vi "NO_SCAN.vi"(8 "stop":bool, 10 "Address Type":T1=1 items=["Public", "Random"], 11 "COM Bluegiga in":refnum<visa-resource-name>="COM13") -> (0 "Reading":bool, 1 "z":dbl, 3 "Connected":bool)   [LabVIEW 2020]
uses:
  <vilib>/BLE/type_def/connection_status_bundle.ctl
  <vilib>/BLE/type_def/address_type.ctl
panel:
  out "w":dbl
  out "x":dbl
  out "y":dbl
  out "characteristic value":u8[](array[numeric])
  out "MAC Address":string
  in  "Service UUID":string="EF6802009B3549339B1052FFA9740042"
  in  "Characteristic UUID":string="EF6802019B3549339B1052FFA9740042"
  out "Handle table":string[][](array[string])
  out "Connection Status":T2={"MAC Address"="", "cnx handle"=0, "cnx flags"=0, "Address Type"=125, "Connection Interval (ms)"=125, "Timeout(ms)"=125, "Latency"=0, "bonding handle"=0} {"Address Type" items=["Public", "Random"]}
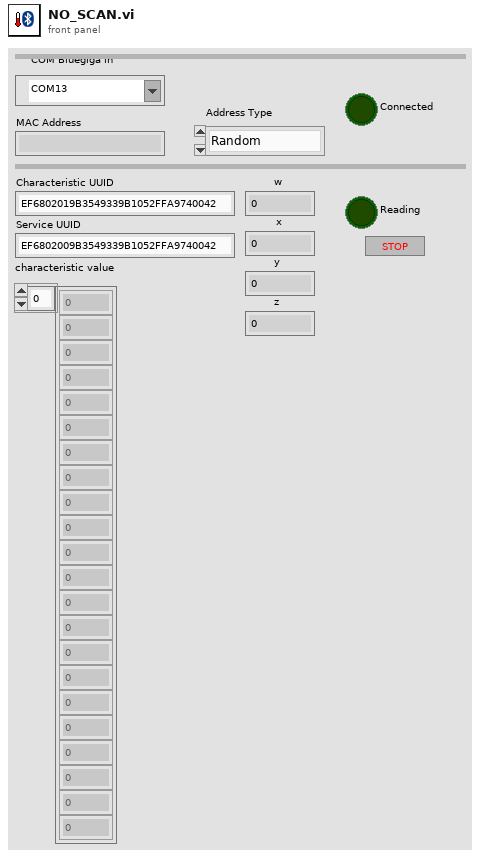
[diagram p1: front panel]
types:
  T1 = typedef "address_type.ctl" = u8
  T2 = typedef "connection_status_bundle.ctl" = cluster{"MAC Address":string, "cnx handle":u8, "cnx flags":u8, "Address Type":T1, "Connection Interval (ms)":u16, "Timeout(ms)":u16, "Latency":u16, "bonding handle":u8}
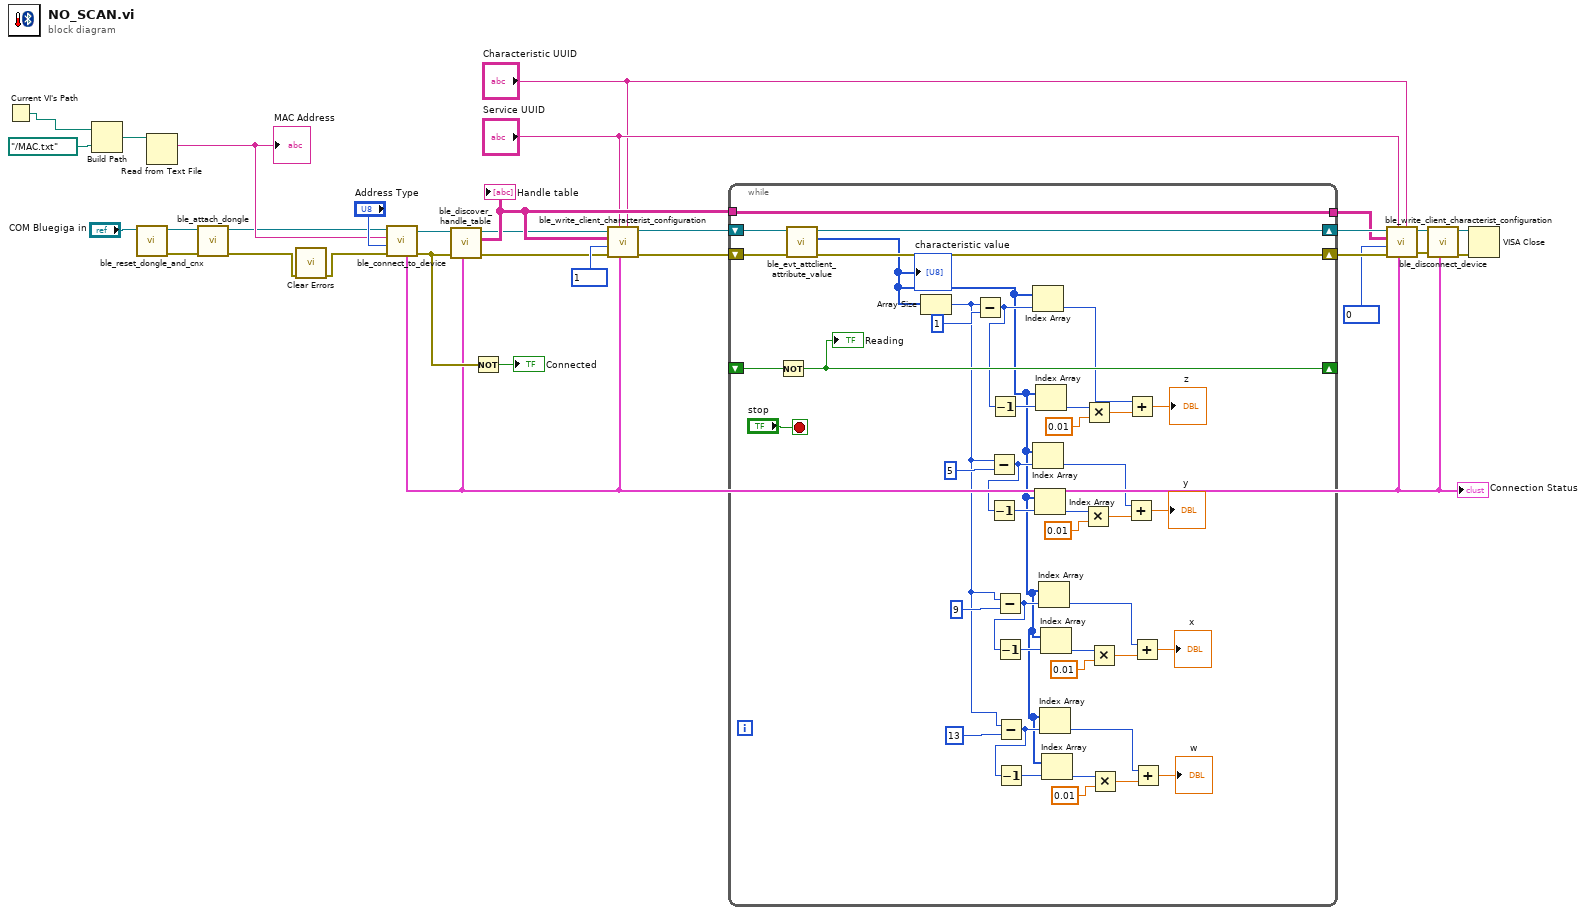
[diagram p0: block diagram]
diagram:
  n1 = Current VI's Path() -> (path=w4:path)
  n2 = Build Path(base path=w4, name or relative path=path "../MAC.txt") -> (appended path=w5:path)
  n3 = call <vilib>:"ble_reset_dongle_and_cnx.vi"("COM Bluegiga in"="COM Bluegiga in") -> ("error out"=w29:errorcluster, "COM Bluegiga out"=w27:refnum<visa-resource-name>)  [unwired: 9 in]
  n4 = Read from Text File(file (use dialog)=w5) -> (text=w7:string)  [unwired: 3 in, 3 out]
  "MAC Address" <- w7
  n5 = call <vilib>:"ble_attach_dongle.vi"("error in (no error)"=w29, "COM Bluegiga in"=w27) -> ("error out"=w2:errorcluster, "COM Bluegiga out"=w3:refnum<visa-resource-name>)  [unwired: 8 in]
  n6 = call <vilib>:"Clear Errors.vi"("error in (no error)"=w2) -> ("error out"=w9:errorcluster)  [unwired: 5 in, 1 out]
  n7 = call <vilib>:"ble_connect_to_device.vi"("Address Type"="Address Type", "error in (no error)"=w9, "MAC Address"=w7, "COM Bluegiga in"=w3) -> ("error out"=w25:errorcluster, "COM Bluegiga out"=w26:refnum<visa-resource-name>, "Connection Status"=w19:T2)  [unwired: 5 in]
  "Connection Status" <- w19
  n8 = call <vilib>:"ble_discover_handle_table.vi"("Connection Status"=w19, "error in (no error)"=w25, "COM Bluegiga in"=w26) -> ("error out"=w14:errorcluster, "Handle table"=w16:string[][], "COM Bluegiga out"=w15:refnum<visa-resource-name>)  [unwired: 6 in]
  "Handle table" <- w16
  n9 = Not(x=w25) -> (.not. x?=→"Connected":bool)
  n10 = call <vilib>:"ble_write_client_characterist_configuration.vi"("Characteristic UUID"="Characteristic UUID", "Connection Status"=w19, "Service UUID"="Service UUID", "error in (no error)"=w14, "Value(16bit)"=u16 1, "Handle table"=w16, "COM Bluegiga in"=w15) -> ("error out"=w12:errorcluster, "COM Bluegiga out"=w13:refnum<visa-resource-name>)  [unwired: 3 in]
  n11 = while {
    tunnel: w16 -> [w68]
    shift-right: [w71] -> w23
    shift-left: w13 -> [w73]
    shift-right: [w67] -> w24
    shift-left: w12 -> [w72]
    tunnel: [w68] -> w22
    shift-right: [w70] -> _
    shift-left: _ -> [w69]
    stop <- "stop" stop-if-true
    n12 = Not(x=w69) -> (.not. x?=w70:bool)
    "Reading" <- w70
    n13 = call <vilib>:"ble_evt_attclient_attribute_value.vi"("error in (no error)"=w72, "COM Bluegiga in"=w73) -> ("error out"=w67:errorcluster, "characteristic value"=w33:u8[], "COM Bluegiga out"=w71:refnum<visa-resource-name>)  [unwired: 6 in, 1 out]
    "characteristic value" <- w33
    n14 = Array Size(array=w33) -> (size(s)=w32:i32)
    n15 = Subtract(x=w32, y=1) -> (x-y=w58:i32)
    n16 = Subtract(x=w32, y=5) -> (x-y=w52:i32)
    n17 = Decrement(x=w52) -> (x-1=w57:i32)
    n18 = Decrement(x=w58) -> (x-1=w64:i32)
    n19 = Subtract(x=w32, y=9) -> (x-y=w44:i32)
    n20 = Decrement(x=w44) -> (x-1=w49:i32)
    n21 = Subtract(x=w32, y=13) -> (x-y=w36:i32)
    n22 = Decrement(x=w36) -> (x-1=w41:i32)
    n23 = Index Array(array=w33, index=w58) -> (element=w60:u8)
    n24 = Index Array(array=w33, index=w52) -> (element=w50:u8)
    n25 = Index Array(array=w33, index=w57) -> (element=w51:u8)
    n26 = Index Array(array=w33, index=w64) -> (element=w63:u8)
    n27 = Index Array(array=w33, index=w44) -> (element=w42:u8)
    n28 = Index Array(array=w33, index=w36) -> (element=w34:u8)
    n29 = Index Array(array=w33, index=w49) -> (element=w43:u8)
    n30 = Index Array(array=w33, index=w41) -> (element=w35:u8)
    n31 = Multiply(x=w51, y=0.01) -> (x*y=w55:dbl)
    n32 = Multiply(x=w63, y=0.01) -> (x*y=w61:dbl)
    n33 = Multiply(x=w43, y=0.01) -> (x*y=w47:dbl)
    n34 = Multiply(x=w35, y=0.01) -> (x*y=w39:dbl)
    n35 = Add(x=w50, y=w55) -> (x+y=→"y":dbl)
    n36 = Add(x=w60, y=w61) -> (x+y=→"z":dbl)
    n37 = Add(x=w42, y=w47) -> (x+y=→"x":dbl)
    n38 = Add(x=w34, y=w39) -> (x+y=→"w":dbl)
  }
  n39 = call <vilib>:"ble_write_client_characterist_configuration.vi"("Characteristic UUID"="Characteristic UUID", "Connection Status"=w19, "Service UUID"="Service UUID", "error in (no error)"=w24, "Value(16bit)"=u16 0, "Handle table"=w22, "COM Bluegiga in"=w23) -> ("error out"=w20:errorcluster, "COM Bluegiga out"=w21:refnum<visa-resource-name>)  [unwired: 3 in]
  n40 = call <vilib>:"ble_disconnect_device.vi"("Connection Status"=w19, "error in (no error)"=w20, "COM Bluegiga in"=w21) -> ("error out"=w30:errorcluster, "COM Bluegiga out"=w31:refnum<visa-resource-name>)  [unwired: 7 in]
  n41 = VISA Close(VISA resource name=w31, error in (no error)=w30) -> ()  [unwired: 1 out]
